vi "Compass Calibrate.vi"() -> ()   [LabVIEW 2012]
uses:
  <vilib>/Platform/TimedLoop/XDataNode/timing_clust.ctl
  <vilib>/Platform/TimedLoop/XDataNode/nitl_modes.ctl
  <vilib>/Platform/TimedLoop/XDataNode/wakeup.ctl
  <vilib>/FPGAPlugInAG/sbRIO-9636/niLvFpga_Open_sbRIO-9636.vi
  <vilib>/rvi/interface/common/dynamic/niFpgaDynamicAddResources.vi
  <vilib>/FPGAPlugInAG/Dynamic/niLvFpga_Close_Dynamic.vi
  <vilib>/platform/TimedLoop/XDataNode/XDataNode.xnode
  <vilib>/rvi/interface/nirviOpenFPGA/nirviOpenFPGA.xnode
  FPGA Bitfiles/NIARC_FPGATarget_FPGACompile_e4XhunWUay0.lvbitx
  <vilib>/rvi/interface/nirviCloseFPGA/nirviCloseFPGA.xnode
  Compass IO.lvlib
  <vilib>/IEDriver/SPIandI2C/Host/I2C/I2C Host.lvlib
  <vilib>/Platform/TimedLoop/XDataNode/XDNodeRunTimeDep.lvlib
panel:
  in  "Enable":bool
  in  "Robot Velocities":T1 {"Angular Velocity (rad/s)" min=-1.0 max=1.0 scale=1.0..-1.0; "Y Velocity (m/s)" min=-1.0 max=1.0 scale=-1.0..1.0; "X Velocity (m/s)" min=-1.0 max=1.0 scale=-1.0..1.0}
  in  "stop":bool
  out "Time":dbl
  in  "Stop":bool
  in  "Start":bool
  # "COMPASS CALIBRATION ROUTINE\n=======================\nPress START and rotate compass 3 times over 30 seconds,\nthen press stop."
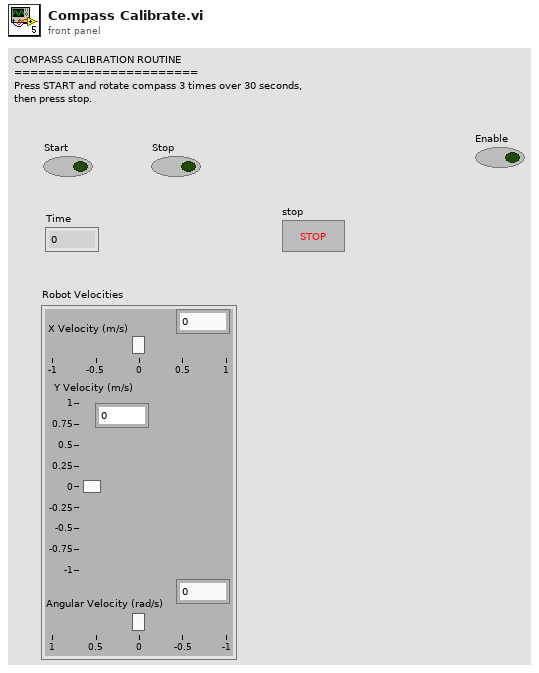
[diagram p1: front panel]
types:
  T1 = cluster{"X Velocity (m/s)":dbl, "Y Velocity (m/s)":dbl, "Angular Velocity (rad/s)":dbl}
  T2 = cluster{"FPGA VI Reference":refnum<k20>, "Port Number":u8}
  T3 = typedef "XDNodeRunTimeDep.lvlib/timing_clust.ctl" = cluster{"Expected End [f-1]":u64, "Actual End [f-1]":u64, "Finished Late? [f-1]":bool, "Expected End [i-1]":u64, "Actual End [i-1]":u64, "Finished Late? [i-1]":bool, "Expected Start [i]":u64, "Actual Start [i]":u64, "Expected Start [f]":u64, "Actual Start [f]":u64, "Source Name":string, "Structure Name":string, "Period":i64, "Deadline":i64, "Offset":i64, "Start":i64, "Priority":i32, "Timeout":i32, "Mode":T4, "Wakeup Reason":T5, "Error":errorcluster, "Source Type":string, "Secondary Source Type":string, "Global End Time":u64, "Global Start Time":u64, "Frame Duration":u64, "Iteration Duration":u64, "Assigned CPU":i32, "I/O Scan Engine Mode":u32}
  T4 = typedef "XDNodeRunTimeDep.lvlib/nitl_modes.ctl" = enum32{"No Change", "Process missed periods, maintain original phase", "Discard missed periods, maintain original phase", "Process missed periods, ignore original phase", "Discard missed periods, ignore original phase"}
  T5 = typedef "XDNodeRunTimeDep.lvlib/wakeup.ctl" = enum32{"Normal", "Aborted", "Asynchronous wakeup", "Timing source error", "Timed loop error", "Timeout"}
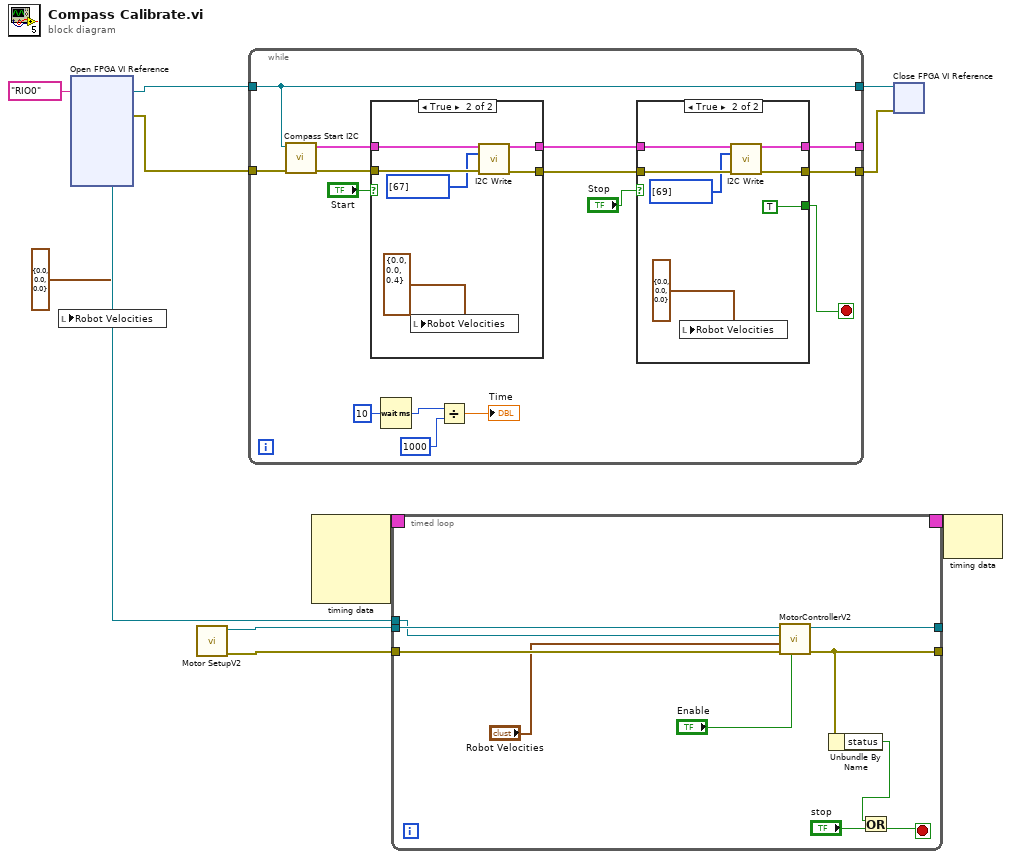
[diagram p0: block diagram]
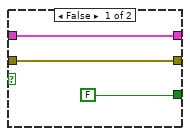
[diagram p2: hidden frame]
diagram:
  n1 = local write "Robot Velocities"(T1 {"X Velocity (m/s)"=0.0, "Y Velocity (m/s)"=0.0, "Angular Velocity (rad/s)"=0.0} ("Robot Velocities")) -> ()
  n2 = xnode "Open FPGA VI Reference"("resource name"=tag "RIO0") -> ("FPGA VI Reference Out"=w2:refnum<k20>, "error out"=w7:errorcluster)  [unwired: 1 in]
  n3 = call "Motor SetupV2.vi"() -> ("error out"=w3:errorcluster, "mecanum steering frame out"=w4:refnum<class "NI_Robotics_Mecanum Steering Frame.lvclass">)  [unwired: 10 in]
  n4 = while {
    tunnel: [w23] -> _
    tunnel: w2 -> [w16]
    tunnel: [w16] -> w10
    tunnel: [w21] -> w8
    tunnel: w7 -> [w15]
    stop <- w19 stop-if-true
    n5 = call "Compass Start I2C.vi"("error in (no error)"=w15, "Refnum in"=w16) -> ("error out"=w17:errorcluster, "FPGA Information Out"=w18:T2)  [unwired: 8 in]
    n6 = case shown="True" "Start" {
      tunnel: w18 -> [w37 w43]
      tunnel: [w37 w42] -> w24
      tunnel: w17 -> [w36 w41]
      tunnel: [w36 w40] -> w22
      frame False {
      }
      frame True {
        n7 = local write "Robot Velocities"(T1 {"X Velocity (m/s)"=0.0, "Y Velocity (m/s)"=0.0, "Angular Velocity (rad/s)"=0.4} ("Robot Velocities")) -> ()
        n8 = call <vilib>:"I2C Write.vi"("FPGA Information In"=w43, "Data"=u8[] [67], "error in (no error)"=w41) -> ("FPGA Information Out"=w42:T2, "error out"=w40:errorcluster)  [unwired: 11 in]
      }
    }
    n9 = Wait (ms)(milliseconds to wait=u32 10) -> (millisecond timer value=w12:u32)
    n10 = Divide(x=w12, y=u32 1000) -> (x/y=→"Time":dbl)
    n11 = case shown="True" "Stop" {
      tunnel: w24 -> [w28 w35]
      tunnel: [w28 w34] -> w23
      tunnel: w22 -> [w27 w33]
      tunnel: [w27 w32] -> w21
      tunnel: [FALSE TRUE] -> w19
      frame False {
      }
      frame True {
        n12 = local write "Robot Velocities"(T1 {"X Velocity (m/s)"=0.0, "Y Velocity (m/s)"=0.0, "Angular Velocity (rad/s)"=0.0} ("Robot Velocities")) -> ()
        n13 = call <vilib>:"I2C Write.vi"("FPGA Information In"=w35, "Data"=u8[] [69], "error in (no error)"=w33) -> ("FPGA Information Out"=w34:T2, "error out"=w32:errorcluster)  [unwired: 11 in]
      }
    }
  }
  n14 = node-c288() -> (w6:T3)  [unwired: 4 in]
  n15 = timed-loop {
    timing: w6 -> [_]
    timing-out: [_] -> w5
    tunnel: w4 -> [w53]
    tunnel: w3 -> [w52]
    tunnel: [w47] -> _
    tunnel: [w51] -> _
    tunnel: w2 -> [w50]
    stop <- w48 stop-if-true
    n16 = call "MotorControllerV2.vi"("Enable"="Enable", "error in"=w52, "Robot Velocities"="Robot Velocities", "FPGA VI Reference In"=w50, "mecanum steering frame in"=w53) -> ("error out"=w47:errorcluster, "steering frame out"=w51:refnum<class "NI_Robotics_Mecanum Steering Frame.lvclass">)  [unwired: 5 in]
    n17 = Unbundle By Name(w47) -> ("status"=w46:bool)
    n18 = Or(x=w46, y="stop") -> (x .or. y?=w48:bool)
  }
  n19 = xnode "Close FPGA VI Reference"("FPGA VI Reference In"=w10, "error in"=w8) -> ()  [unwired: 1 out]
  n20 = node-c288(w5) -> ()  [unwired: 1 out]
